vi "Resample Waveforms.vi"(8 "error in":errorcluster, 9 "pd resample Factor":i32=2, 10 "time resample Factor":i32=5, 11 "PAS Cell Data in":refnum<class "PAS Cell Data.lvclass">) -> (0 "error out":errorcluster, 3 "PAS Cell Data out":refnum<class "PAS Cell Data.lvclass">)   [LabVIEW 2017, in "PAS Library.lvlib" / "PAS Cell Data.lvclass"]
doc: "Resampe the waveforms for transmission and display by the host."
uses:
  PAS Cell Data.lvclass
  PAS Cell Data.lvclass/PAS Cell Data.ctl
  <vilib>/Waveform/WDTOps.llb/WDT Get Waveform Subset SGL.vi
  <vilib>/measure/maresamp.llb/Resample Waveform (continuous).vi
  <vilib>/measure/NI_MAPro.lvlib
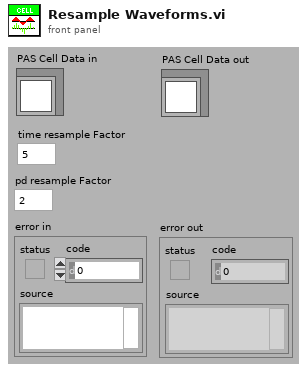
[diagram p1: front panel]
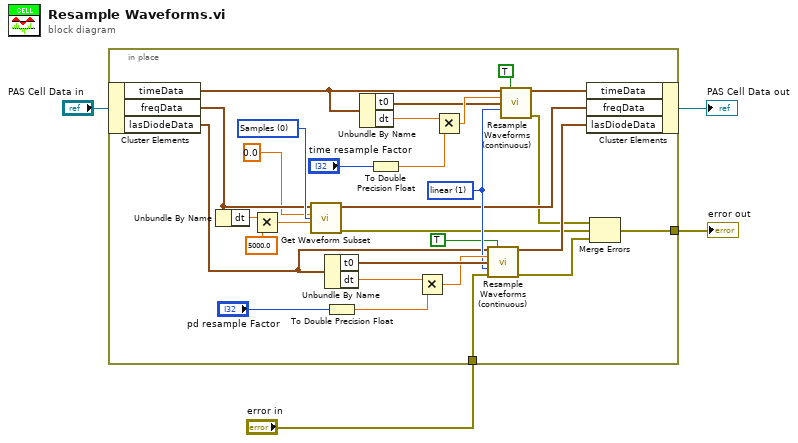
[diagram p0: block diagram]
diagram:
  n1 = in-place {
    in-place-border: [w15] -> w4
    in-place-border: "error in" -> [w11]
    w23 = u16 0 items=["Samples", "Relative Time"] ("start/duration format")
    w24 = u16 1 items=["coerce", "linear", "spline", "FIR filter"] ("interpolation mode")
    n2 = in-place-cluster #1("PAS Cell Data in") -> ("timeData"=w14:waveform(i16), "freqData"=w21:waveform(sgl), "lasDiodeData"=w13:waveform(i16))
    n3 = Unbundle By Name(w21) -> ("dt"=w31:dbl)
    n4 = Multiply(x=w31, y=5000.0) -> (x*y=w32:dbl)
    n5 = call-poly <vilib>:"Get Waveform Subset.vi"("start/duration format"=w23, "duration"=w32, "start samples/time"=0.0, "waveform in"=w21) -> ("error out"=w17:errorcluster, "waveform out"=w20:waveform(sgl))  [unwired: 2 in, 2 out]
    n6 = Unbundle By Name(w13) -> ("t0"=w26:timestamp, "dt"=w8:dbl)
    n7 = To Double Precision Float(number="pd resample Factor") -> (double precision float=w5:dbl)
    n8 = Unbundle By Name(w14) -> ("t0"=w27:timestamp, "dt"=w29:dbl)
    n9 = To Double Precision Float(number="time resample Factor") -> (double precision float=w9:dbl)
    n10 = Multiply(x=w8, y=w5) -> (x*y=w25:dbl)
    n11 = Multiply(x=w29, y=w9) -> (x*y=w28:dbl)
    n12 = call-poly <vilib>:"Resample Waveforms (continuous).vi"("waveform in"=w13, "reset"=TRUE, "dt"=w25, "t0"=w26, "interpolation mode"=w24, "error in (no error)"=w11) -> ("resampled waveform out"=w19:waveform(dbl), "error out"=w16:errorcluster)  [unwired: 5 in, 3 out]
    n13 = call-poly <vilib>:"Resample Waveforms (continuous).vi"("waveform in"=w14, "reset"=TRUE, "dt"=w28, "t0"=w27, "interpolation mode"=w24) -> ("resampled waveform out"=w22:waveform(dbl), "error out"=w18:errorcluster)  [unwired: 6 in, 3 out]
    n14 = in-place-cluster #1("timeData"=w22, "freqData"=w20, "lasDiodeData"=w19) -> (→"PAS Cell Data out":refnum<class "PAS Cell Data.lvclass">)
    n15 = Merge Errors(w18, w17, w16) -> (w15:errorcluster)
  }
  "error out" <- w4
